vi "Read Sample Containers.vi"(11 "Sample Line in":refnum<class "Sample Line.lvclass">) -> (2 "Sample Containers":T1[](array[typedef])=[{"Sample In"="ni.var.psp://localhost/AMS Gas SHV/Sample Lines/Line 1/Sample In", "Sample Name"="ni.var.psp://localhost/AMS Gas SHV/Sample Lines/Line 1/Sample Name", "Ti Cathode"="ni.var.psp://localhost/AMS Gas SHV/Sample Lines/Line 1/Ti Cathode", "SampleQ"=refnum}, {"Sample In"="ni.var.psp://localhost/AMS Gas SHV/Sample Lines/Line 2/Sample In", "Sample Name"="ni.var.psp://localhost/AMS Gas SHV/Sample Lines/Line 2/Sample Name", "Ti Cathode"="ni.var.psp://localhost/AMS Gas SHV/Sample Lines/Line 2/Ti Cathode", "SampleQ"=refnum}, {"Sample In"="ni.var.psp://localhost/AMS Gas SHV/Sample Lines/Line 3/Sample In", "Sample Name"="ni.var.psp://localhost/AMS Gas SHV/Sample Lines/Line 3/Sample Name", "Ti Cathode"="ni.var.psp://localhost/AMS Gas SHV/Sample Lines/Line 3/Ti Cathode", "SampleQ"=refnum}, {"Sample In"="ni.var.psp://localhost/AMS Gas SHV/Sample Lines/Line 4/Sample In", "Sample Name"="ni.var.psp://localhost/AMS Gas SHV/Sample Lines/Line 4/Sample Name", "Ti Cathode"="ni.var.psp://localhost/AMS Gas SHV/Sample Lines/Line 4/Ti Cathode", "SampleQ"=refnum}, {"Sample In"="ni.var.psp://localhost/AMS Gas SHV/Sample Lines/Line 5/Sample In", "Sample Name"="ni.var.psp://localhost/AMS Gas SHV/Sample Lines/Line 5/Sample Name", "Ti Cathode"="ni.var.psp://localhost/AMS Gas SHV/Sample Lines/Line 5/Ti Cathode", "SampleQ"=refnum}], 3 "Sample Line out":refnum<class "Sample Line.lvclass">)   [LabVIEW 2015, in "cRIO-Carbondioxide.lvlib" / "CO2-Actor.lvlib" / "Sample Line.lvclass"]
uses:
  Sample Line.lvclass
  Controls/Sample Container.ctl
  subs/Sample/Sample.lvclass
  Sample Line.lvclass/Sample Line.ctl
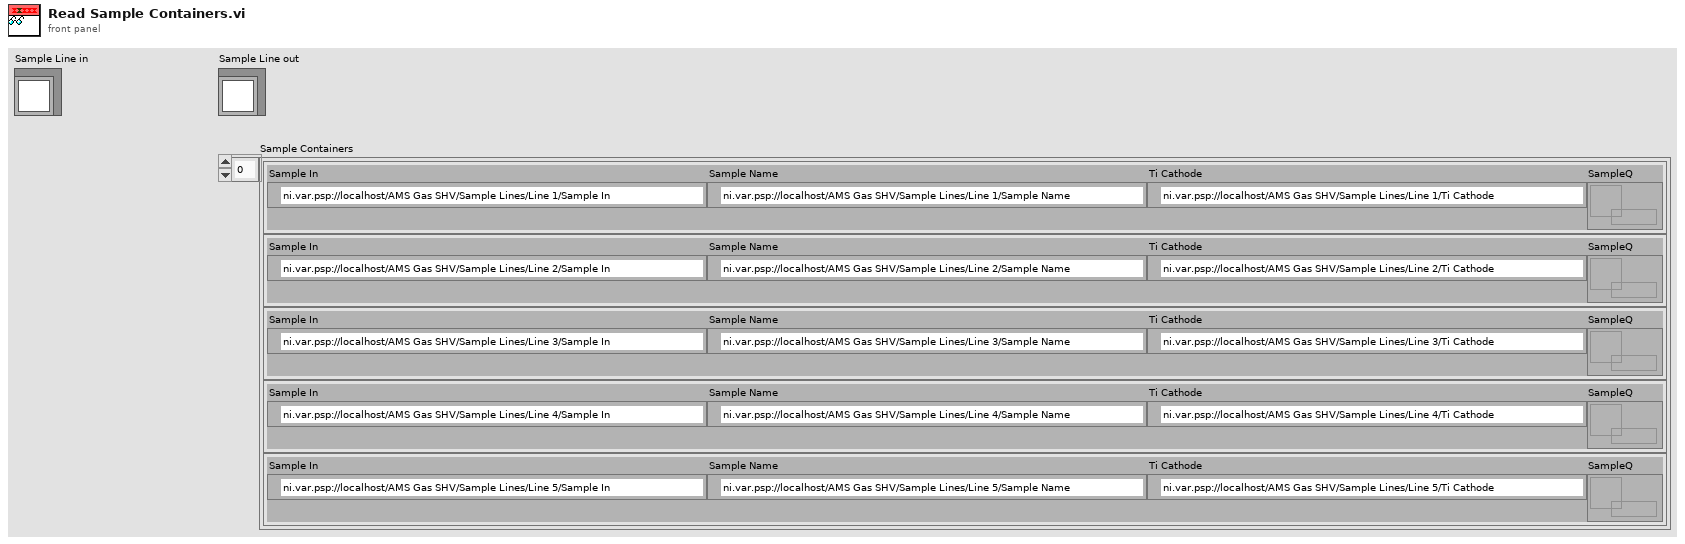
[diagram p1: front panel]
types:
  T1 = typedef "Sample Container.ctl" = cluster{"Sample In":refnum<k21>, "Sample Name":refnum<k21>, "Ti Cathode":refnum<k21>, "SampleQ":refnum<queue>}
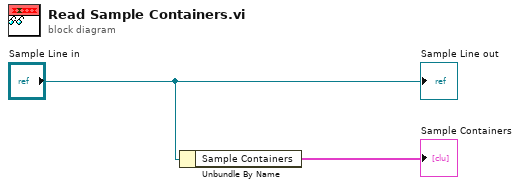
[diagram p0: block diagram]
diagram:
  n1 = Unbundle By Name("Sample Line in") -> ("Sample Containers"=→"Sample Containers":T1[])
  "Sample Line out" <- "Sample Line in"
